vi "chart series get error bars.vi"(8 "error in (no error)":errorcluster, 10 "axis_type":u8, 11 "series":u32) -> (0 "error out":errorcluster, 3 "function return":u32)   [LabVIEW 2015, in "xlsxwriter.lvlib"]
doc: "lxw_series_error_bars chart_series_get_error_bars(lxw_chart_series series, uint8_t axis_type);"
uses:
  xlsxwriter.lvlib
  xlsxwriter.dll
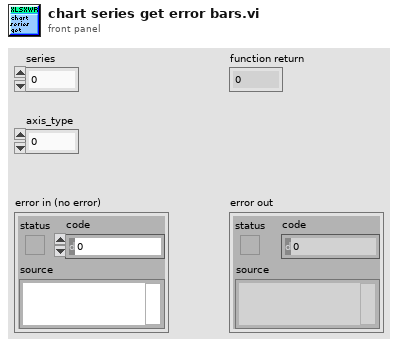
[diagram p1: front panel]
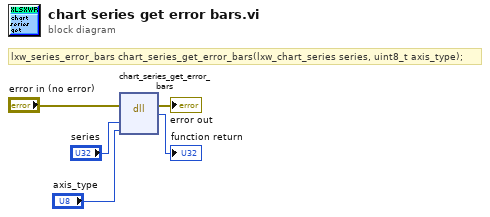
[diagram p0: block diagram]
diagram:
  # "lxw_series_error_bars chart_series_get_error_bars(lxw_chart_series series, uint8_t axis_type);"
  n1 = dll-call lib="C:/Users/WDAGUtilityAccount/Desktop/lv_vis_added_cell/xlsxwriter.*" fn="chart_series_get_error_bars"(error in="error in (no error)", "series"="series", "axis_type"="axis_type") -> (error out=→"error out":errorcluster, →"function return":u32)  [unwired: 4 in, 1 out]
